vi "poly_search_vis_in_memory_exec_multi.vi"(7 "app ref (open local)":refnum<vi>, 8 "error in (no error)":errorcluster, 9 "additional search items":T2={"+ in lvlibs"=TRUE, " + controls"=FALSE, " + self"=FALSE, "+ instances"=FALSE, "+ in llbs"=TRUE}, 10 "tagert exectution states":T1(array[ring])) -> (0 "error out":errorcluster, 1 "vi paths":path[](array[path]), 2 "vi names":string[](array[string]), 5 "n of vis found":i32)   [LabVIEW 2015]
doc: "Check the execution state of all VIs in the current application (or in the app reference wired <- not tested). \n\nThe target execution states are\n - \"Run Top Level\" - Runnign vi\n - \"Running\" - Running sub vi\n - \"Idle\" - Loaded in memory but not running\n - \"Bad\" - Not executable\n\nYou can use additional search items to also specity whether to search for VIs in\n - lvlibs (T)\n - llbs (T)\n - .ctl files (F)\n - reetnant instances (F)\n - this vi (F)"
uses:
  misc_tools/SearchItems.ctl
  <vilib>/regexp/Match Regular Expression.xnode
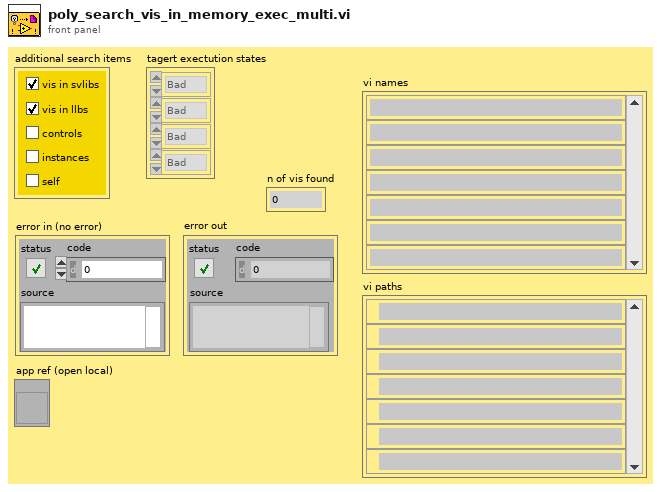
[diagram p1: front panel]
types:
  T1 = enum32{"Bad", "Idle", "Run top level", "Running"}[]
  T2 = typedef "SearchItems.ctl" = cluster{"+ in lvlibs":bool, " + controls":bool, " + self":bool, "+ instances":bool, "+ in llbs":bool}
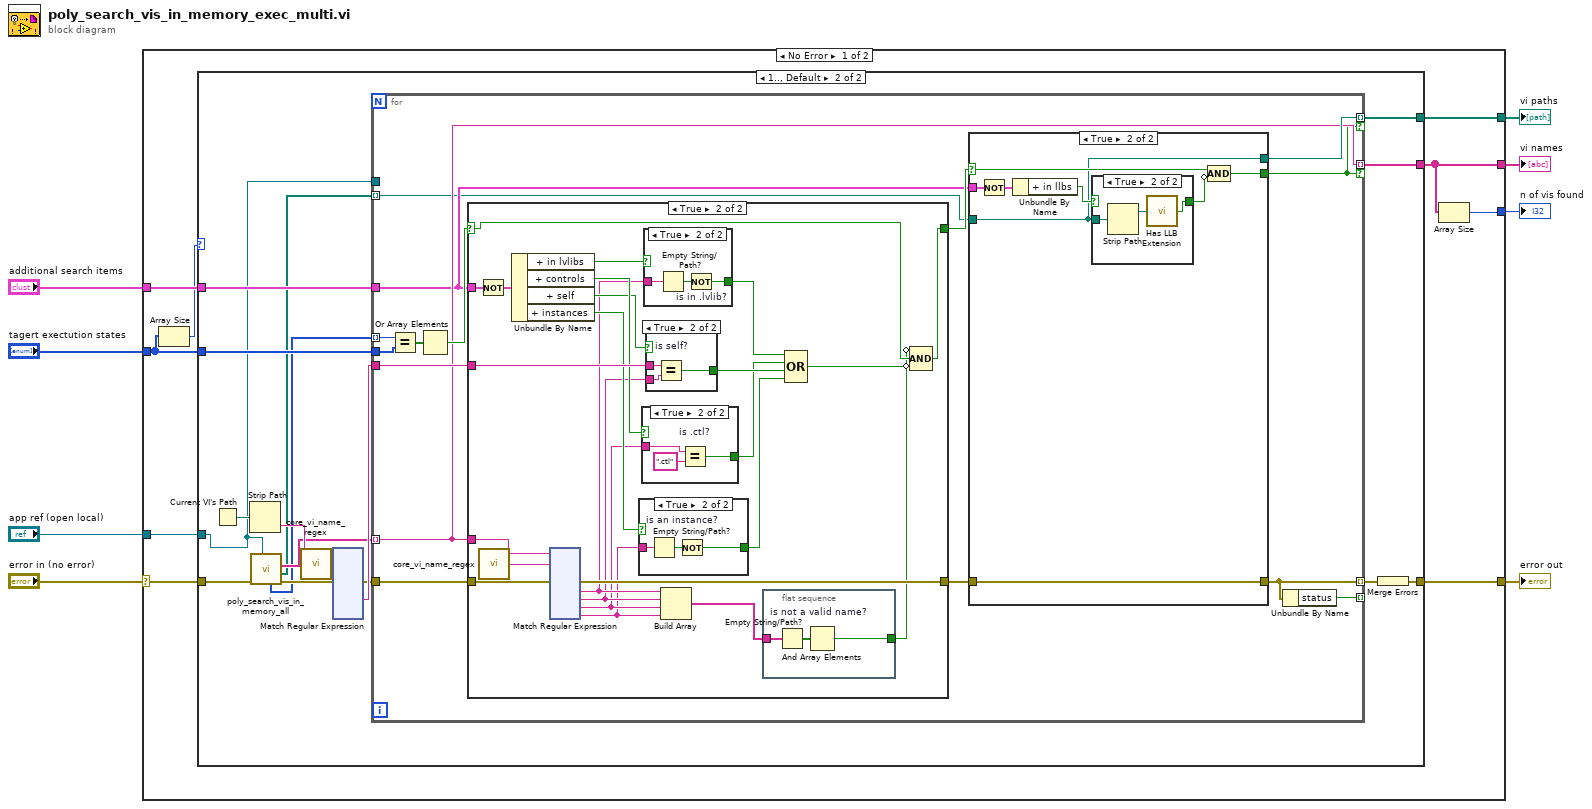
[diagram p0: block diagram]
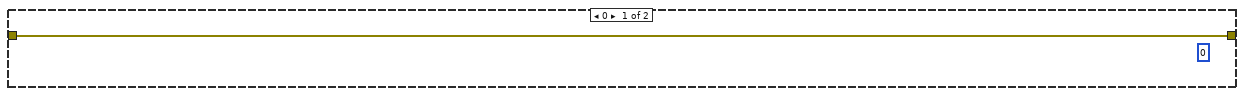
[diagram p2: hidden frame]
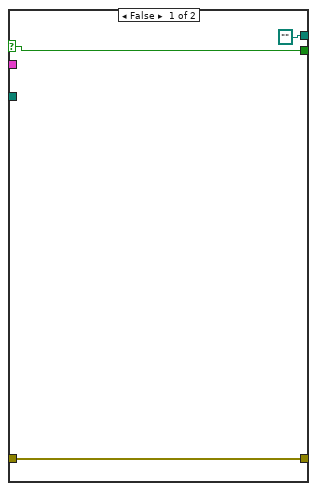
[diagram p3: hidden frame]
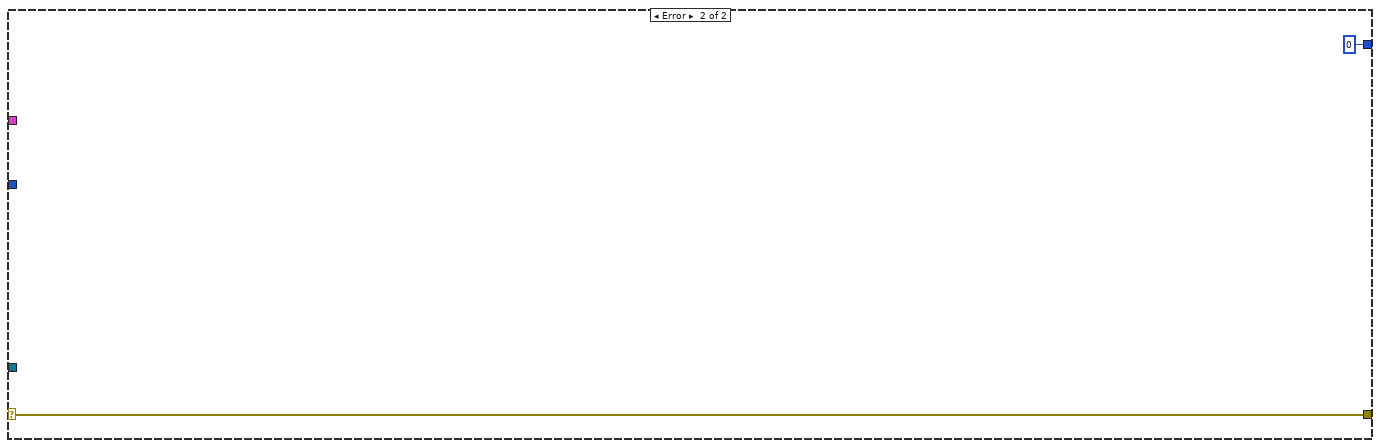
[diagram p10: hidden frame]
diagram:
  n1 = case shown="No Error" "error in (no error)" {
    selector: "error in (no error)" -> [w16 w350]
    tunnel: "additional search items" -> [w15 _]
    tunnel: [w17 w350] -> w7
    tunnel: [w12 0] -> w5
    tunnel: [w14 _] -> w3
    tunnel: [w13 _] -> w4
    tunnel: "tagert exectution states" -> [w11 _]
    tunnel: "app ref (open local)" -> [w9 _]
    frame No Error {
      n2 = Array Size(array=w11) -> (size(s)=w10:i32)
      n3 = case shown="1.., Default" w10 {
        tunnel: w16 -> [w18 w24]
        tunnel: [w18 w21] -> w17
        tunnel: w15 -> [_ w34]
        tunnel: [_ w32] -> w14
        tunnel: [_ w31] -> w13
        tunnel: w11 -> [_ w27]
        tunnel: w9 -> [_ w25]
        frame 0 {
          (unwired) 0
        }
        frame 1.., Default {
          n4 = Current VI's Path() -> (path=w35:path)
          n5 = Strip Path(path=w35) -> (name=w30:string)  [unwired: 1 out]
          n6 = call "poly_search_vis_in_memory_all.vi"("app ref (open local)"=w25, "error in (no error)"=w24) -> ("error out"=w23:errorcluster, "vi paths"=w20:path[], "vi names"=w22:string[], "execution states"=w19:T1)  [unwired: 5 in, 1 out]
          n7 = call "core_vi_name_regex.vi"() -> ("regex"=w26:string)
          n8 = xnode "Match Regular Expression"("input string"=w30, "regular expression"=w26, "error in"=w23) -> ("error out"=w28:errorcluster, "submatch 2"=w29:string)  [unwired: 3 in, 7 out]
          n9 = for {
            tunnel: w22 -> [w164] mode=indexing
            tunnel: w28 -> [w156]
            tunnel: w25 -> [_]
            tunnel: w29 -> [w168]
            tunnel: w34 -> [w158]
            tunnel: [w167] -> w32 mode=indexing if=w159
            tunnel: [w166] -> w33 mode=indexing
            tunnel: [w165] -> _ mode=indexing
            tunnel: [w164] -> w31 mode=indexing if=w159
            tunnel: w27 -> [w161]
            tunnel: w20 -> [w155] mode=indexing
            tunnel: w19 -> [w157] mode=indexing
            n10 = Equal?(x=w157, y=w161) -> (x = y?=w160:bool[])
            n11 = Or Array Elements(Boolean array=w160) -> (logical OR=w169:bool)
            n12 = case shown="True" w169 {
              selector: w169 -> [w186 w200]
              tunnel: [w186 w198] -> w163
              tunnel: w158 -> [_ w205]
              tunnel: w164 -> [_ w210]
              tunnel: w168 -> [_ w209]
              tunnel: w156 -> [w185 w197]
              tunnel: [w185 w196] -> w162
              frame False {
              }
              frame True {
                n13 = Not(x=w205) -> (.not. x?=w204:T2)
                n14 = call "core_vi_name_regex.vi"() -> ("regex"=w187:string)
                n15 = Unbundle By Name(w204) -> ("+ in lvlibs"=w208:bool, "+ controls"=w207:bool, "+ self"=w206:bool, "+ instances"=w195:bool)
                n16 = xnode "Match Regular Expression"("input string"=w210, "regular expression"=w187, "error in"=w197) -> ("error out"=w196:errorcluster, "submatch 1"=w193:string, "submatch 2"=w192:string, "submatch 3"=w191:string, "submatch 4"=w190:string)  [unwired: 3 in, 4 out]
                n17 = case shown="True" w195 {
                  selector: w195 -> [w214 _]
                  tunnel: w190 -> [_ w217]
                  tunnel: [w214 w215] -> w194
                  frame False {
                  }
                  frame True {
                    n18 = Empty String/Path? ("is in .lvlib?")(string/path=w217) -> (empty?=w216:bool)
                    n19 = Not "is an instance?"(x=w216) -> (.not. x?=w215:bool)
                  }
                }
                n20 = case shown="True" w207 {
                  selector: w207 -> [w226 _]
                  tunnel: [w226 w228] -> w201
                  tunnel: w191 -> [_ w227]
                  frame False {
                  }
                  frame True {
                    n21 = Equal? "is .ctl?"(x=w227, y=".ctl") -> (x = y?=w228:bool)
                  }
                }
                n22 = case shown="True" w208 {
                  selector: w208 -> [w218 _]
                  tunnel: w193 -> [_ w221]
                  tunnel: [w218 w219] -> w203
                  frame False {
                  }
                  frame True {
                    n23 = Empty String/Path? ("is in .lvlib?")(string/path=w221) -> (empty?=w220:bool)
                    n24 = Not "is in .lvlib?"(x=w220) -> (.not. x?=w219:bool)
                  }
                }
                n25 = case shown="True" w206 {
                  selector: w206 -> [w222 _]
                  tunnel: w209 -> [_ w225]
                  tunnel: [w222 w223] -> w202
                  tunnel: w192 -> [_ w224]
                  frame False {
                  }
                  frame True {
                    n26 = Equal? "is self?"(x=w225, y=w224) -> (x = y?=w223:bool)
                  }
                }
                n27 = Build Array(w193, w192, w191, w190) -> (w189:string[])
                n28 = flat-sequence {
                  tunnel: w189 -> [w213]
                  tunnel: [w211] -> w188
                  frame #0 {
                    n29 = Empty String/Path? ("is in .lvlib?")(string/path=w213) -> (empty?=w212:bool[])
                    n30 = And Array Elements "is not a valid name?"(Boolean array=w212) -> (logical AND=w211:bool)
                  }
                }
                n31 = Compound Arithmetic op=OR(w203, w201, w202, w194) -> (w199:bool)
                n32 = Compound Arithmetic op=AND(invert w188, w200, invert w199) -> (w198:bool)
              }
            }
            n33 = case shown="True" w163 {
              selector: w163 -> [w170 w177]
              tunnel: w162 -> [w171 w173]
              tunnel: [path "" w174] -> w167
              tunnel: [w171 w173] -> w166
              tunnel: [w170 w175] -> w159
              tunnel: w158 -> [_ w179]
              tunnel: w155 -> [_ w174]
              frame False {
              }
              frame True {
                n34 = Not(x=w179) -> (.not. x?=w180:T2)
                n35 = Unbundle By Name(w180) -> ("+ in llbs"=w178:bool)
                n36 = case shown="True" w178 {
                  selector: w178 -> [w181 _]
                  tunnel: w174 -> [_ w184]
                  tunnel: [w181 w182] -> w176
                  frame False {
                  }
                  frame True {
                    n37 = Strip Path(path=w184) -> (stripped path=w183:path)  [unwired: 1 out]
                    n38 = call <vilib>:"Has LLB Extension.vi"("path"=w183) -> ("path to VI library?"=w182:bool)
                  }
                }
                n39 = Compound Arithmetic op=AND(w177, invert w176) -> (w175:bool)
              }
            }
            n40 = Unbundle By Name(w166) -> ("status"=w165:bool)
          }
          n41 = Merge Errors(w33) -> (w21:errorcluster)
        }
      }
      n42 = Array Size(array=w13) -> (size(s)=w12:i32)
    }
    frame Error {
    }
  }
  "vi names" <- w4
  "error out" <- w7
  "vi paths" <- w3
  "n of vis found" <- w5
